vi "Read Joystick State.vi"(8 "error in (no error)":errorcluster, 11 "Get Joystick State Msg in":refnum<class "Get Joystick State Msg.lvclass">) -> (0 "error out":errorcluster, 2 "Joystick State":T1, 3 "Get Joystick State Msg out":refnum<class "Get Joystick State Msg.lvclass">)   [LabVIEW 2014, in "Joystick.lvlib" / "Get Joystick State Msg.lvclass"]
uses:
  Get Joystick State Msg.lvclass
  Joystick Class/Joystick State.ctl
  Joystick Class/Button State.ctl
  Joystick Class/Axis State.ctl
  Get Joystick State Msg.lvclass/Get Joystick State Msg.ctl
  Joystick Class/Joystick.lvclass
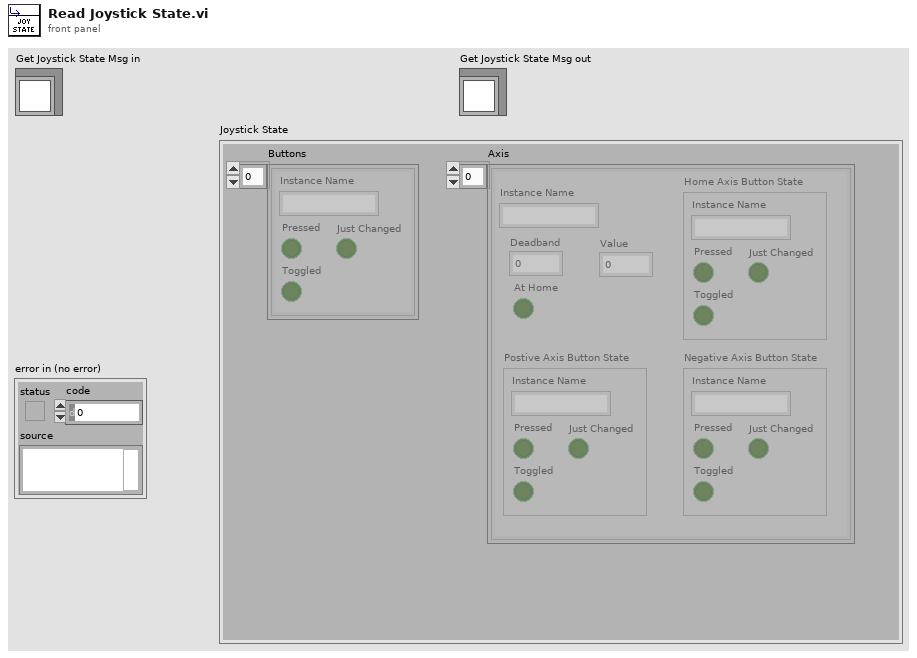
[diagram p1: front panel]
types:
  T1 = typedef "Joystick.lvlib/Joystick.lvclass/Joystick State.ctl" = cluster{"Buttons":T2[], "Axis":T3[]}
  T2 = typedef "Joystick.lvlib/Joystick.lvclass/Button State.ctl" = cluster{"Pressed":bool, "Instance Name":string, "Toggled":bool, "Just Changed":bool}
  T3 = typedef "Joystick.lvlib/Joystick.lvclass/Axis State.ctl" = cluster{"Instance Name":string, "Deadband":dbl, "Value":dbl, "At Home":bool, "Postive Axis Button State":T2, "Negative Axis Button State":T2, "Home Axis Button State":T2}
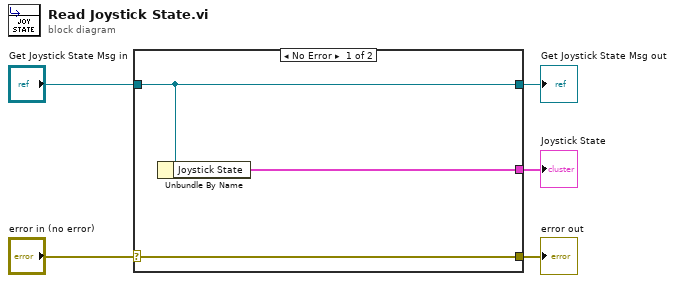
[diagram p0: block diagram]
diagram:
  n1 = case shown="No Error" "error in (no error)" {
    selector: "error in (no error)" -> [w8 w9]
    tunnel: [w8 w9] -> w4
    tunnel: [w7 w10] -> w2
    tunnel: "Get Joystick State Msg in" -> [w7 w10]
    tunnel: [w6 _] -> w1
    frame No Error {
      n2 = Unbundle By Name(w7) -> ("Joystick State"=w6:T1)
    }
    frame Error {
    }
  }
  "error out" <- w4
  "Get Joystick State Msg out" <- w2
  "Joystick State" <- w1
